vi "Test Initiate.vi"(0 "Template Tx Test in":refnum<class "niDTS Calibration Cal Execute RF Test.lvclass">, 11 "error in (no error)":errorcluster) -> (4 "Template Tx Test out":refnum<class "niDTS Calibration Cal Execute RF Test.lvclass">, 15 "error out":errorcluster)   [LabVIEW 2015, in "niDTS Utilities.lvlib" / "niDTS Calibration Cal Execute RF Test.lvclass"]
uses:
  niDTS Calibration Cal Execute RF Test.lvclass
  niDTS Calibration Cal Execute RF Test.lvclass/niDTS Calibration Cal Execute RF Test.ctl
  Properties/Calibration Cal Execute Get InstDriver Handle in.vi
  Properties/Calibration Cal Execute RF Test Get Ports.vi
  Properties/Calibration Cal Execute Set Cal Executed.vi
  RiviInstDriver/niRfGeneralSettings/Objects/niRfGeneralSettings.lvclass
  RiviInstDriver/InstDriver/Objects/InstDriver.lvclass
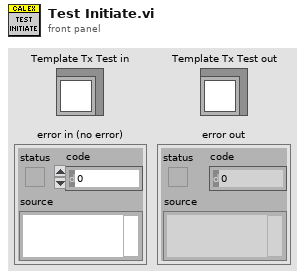
[diagram p1: front panel]
types:
  T1 = typedef "niRfGeneralSettings.lvclass/niRfGeneralSettings INC Handle.ctl" = refnum<data-value>
  T2 = typedef "niDTS Utilities.lvlib/niDTS Calibration Cal Execute RF Test INC Parameters.ctl" = cluster{"Calibration Mode":u16}
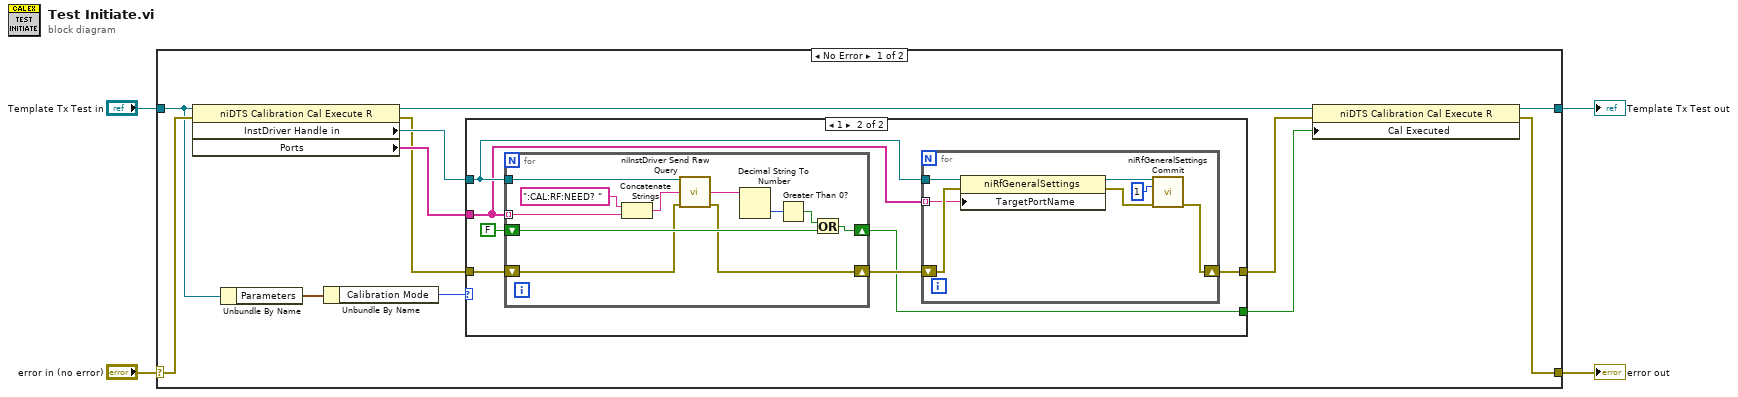
[diagram p0: block diagram]
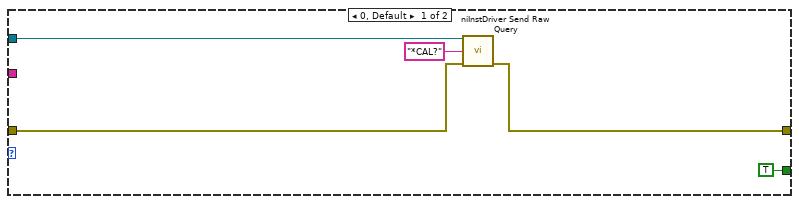
[diagram p2: hidden frame]
diagram:
  n1 = case shown="No Error" "error in (no error)" {
    selector: "error in (no error)" -> [w16 w48]
    tunnel: [w6 w48] -> w3
    tunnel: [w8 w47] -> w1
    tunnel: "Template Tx Test in" -> [w10 w47]
    frame No Error {
      n2 = property class="niDTS Calibration Cal Execute R"(reference=w10, error in=w16) -> (reference out=w9:refnum<class "niDTS Calibration Cal Execute RF Test.lvclass">, error out=w11:errorcluster, "InstDriver Handle in"=w13:T1, "Ports"=w12:string[])
      n3 = Unbundle By Name(w10) -> ("Parameters"=w15:T2)
      n4 = Unbundle By Name(w15) -> ("Calibration Mode"=w14:u16)
      n5 = case shown="1" w14 {
        tunnel: w13 -> [w17 w25]
        tunnel: w12 -> [_ w24]
        tunnel: [w20 w28] -> w7
        tunnel: w11 -> [w18 w27]
        tunnel: [TRUE w23] -> w5
        frame 0, Default {
          n6 = call "niInstDriver Send Raw Query.vi"("InstDriver Handle in"=w17, "Query"="*CAL?" ("Command"), "error in (no error)"=w18) -> ("error out"=w20:errorcluster)  [unwired: 10 in, 2 out]
        }
        frame 1 {
          n7 = for {
            tunnel: w24 -> [w34] mode=indexing
            shift-right: [w32] -> w26
            shift-left: w27 -> [w33]
            shift-right: [w38] -> w23
            shift-left: FALSE -> [w39]
            tunnel: w25 -> [w37]
            n8 = Concatenate Strings(":CAL:RF:NEED? ", w34) -> (w36:string)
            n9 = call "niInstDriver Send Raw Query.vi"("InstDriver Handle in"=w37, "Query"=w36, "error in (no error)"=w33) -> ("Response"=w31:string, "error out"=w32:errorcluster)  [unwired: 10 in, 1 out]
            n10 = Decimal String To Number(string=w31) -> (number=w30:i32)  [unwired: 2 in, 1 out]
            n11 = Greater Than 0?(x=w30) -> (x > 0?=w29:bool)
            n12 = Or(x=w29, y=w39) -> (x .or. y?=w38:bool)
          }
          n13 = for {
            tunnel: w25 -> [w40]
            shift-right: [w41] -> w28
            shift-left: w26 -> [w46]
            tunnel: w24 -> [w45] mode=indexing
            n14 = property class="niRfGeneralSettings"(reference=w40, error in=w46, "TargetPortName"=w45) -> (reference out=w44:T1, error out=w43:errorcluster)
            n15 = call "niRfGeneralSettings Commit.vi"("InstDriver Handle in"=w44, "Instance"=1, "error in (no error)"=w43) -> ("error out"=w41:errorcluster)  [unwired: 11 in, 1 out]
          }
        }
      }
      n16 = property class="niDTS Calibration Cal Execute R"(reference=w9, error in=w7, "Cal Executed"=w5) -> (reference out=w8:refnum<class "niDTS Calibration Cal Execute RF Test.lvclass">, error out=w6:errorcluster)
    }
    frame Error {
    }
  }
  "error out" <- w3
  "Template Tx Test out" <- w1
